vi "Get DTCs From CD and Display.vi"(6 "DTCs":refnum<vi>, 7 "To Top (T)":bool=TRUE, 8 "error in (no error)":errorcluster, 9 "Addresses":refnum<vi>, 10 "Lookup Table In":variant, 11 "connection info":T3) -> (0 "error out":errorcluster, 2 "Lookup Table Out":variant, 3 "connection info":T3, 4 "Error Array":T1[](array[typedef]))   [LabVIEW 2015, in "J1939 Addon Shared.lvlib"]
uses:
  J1939 Addon Shared.lvlib
  <vilib>/NI/STM/TCP/TCP Connection Info.ctl
  <vilib>/NI/STM/SubVIs/MetaDataElement.ctl
  Types/Error Cluster.ctl
  Types/Error Types.ctl
  <vilib>/Utility/miscctls.llb/LVRowAndColumnUnsignedTypeDef.ctl
  <vilib>/NI/STM/NI STM.lvlib
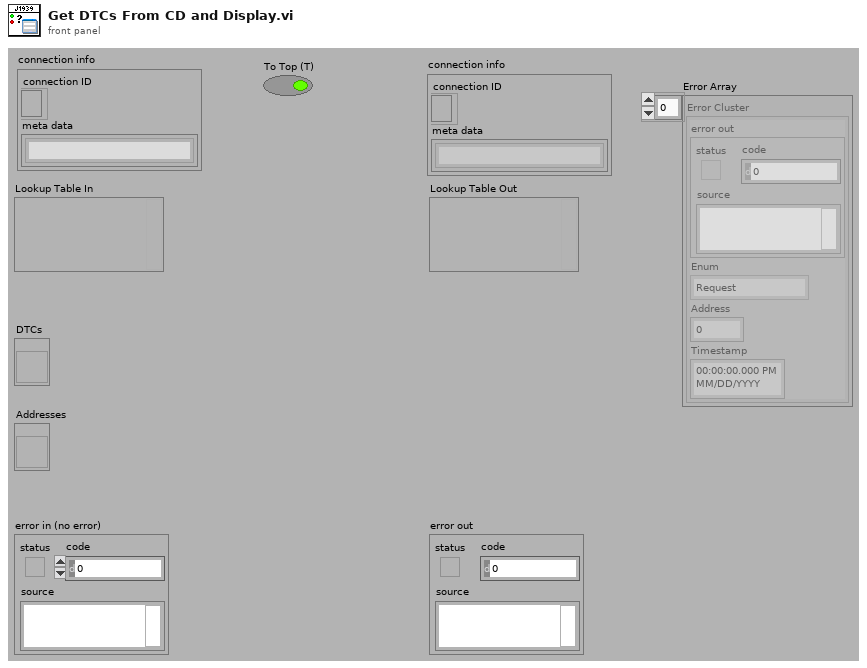
[diagram p1: front panel]
types:
  T1 = typedef "J1939 Addon Shared.lvlib/Error Cluster.ctl" = cluster{"error out":errorcluster, "Enum":T2, "Address":u8, "Timestamp":timestamp}
  T2 = typedef "J1939 Addon Shared.lvlib/Error Types.ctl" = enum16{"Request", "RAW Generation", "Clear Active DTCs", "Clear Previous DTCs", "Addresses", "TLAs", "Get Active DTCs", "Get Previous DTCs"}
  T3 = typedef "NI STM.lvlib/TCP Connection Info.ctl" = cluster{"connection ID":refnum<k5>, "meta data":T4[]}
  T4 = typedef "NI STM.lvlib/MetaDataElement.ctl" = string
  T5 = typedef "J1939 Addon Shared.lvlib/Address Parse Tree Cluster.ctl" = cluster{"Parent Selection":string, "Address Selection":string, "CMD Selection":string}
  T6 = typedef "J1939 Addon Shared.lvlib/Convert DTCs Cluster.ctl" = cluster{"Lamps":cluster{"Protect Lamp":u8, "Amber Warning":u8, "Red Stop":u8, "Malfunction Indicator":u8}, "DTCs":cluster{"SPN":u32, "FMI":u8, "Occurrance":u8}[], "Active?":bool, "Address":u8, "timestamp":timestamp}
  T7 = typedef "LVRowAndColumnUnsignedTypeDef.ctl" = cluster{"Row":u32, "Column":u32}
  T8 = cluster{"Protect Lamp":u8, "Amber Warning":u8, "Red Stop":u8, "Malfunction Indicator":u8}
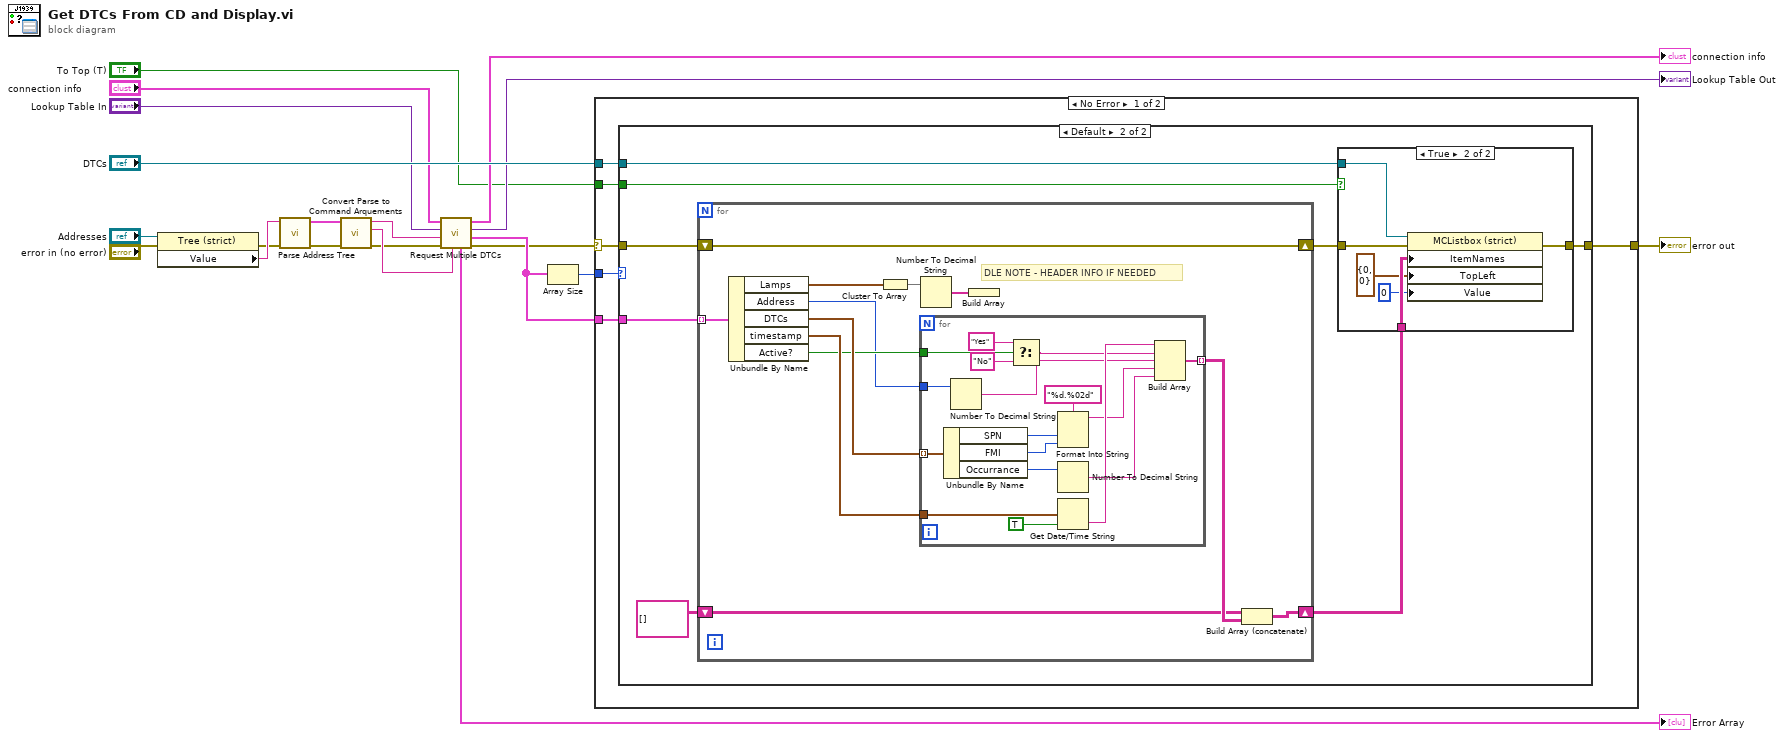
[diagram p0: block diagram]
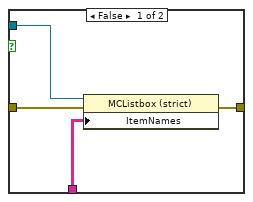
[diagram p3: hidden frame]
diagram:
  n1 = property on="Property Node" class="Tree (strict)"(reference="Addresses", error in="error in (no error)") -> (error out=w14:errorcluster, "Value"=w15:string)  [unwired: 1 out]
  n2 = call "Parse Address Tree.vi"("error in"=w14, "Address Selection"=w15) -> ("error out"=w5:errorcluster, "Address Parsed Tree"=w16:T5)  [unwired: 8 in]
  n3 = call "Convert Parse to Command Arquements.vi"("error in (no error)"=w5, "Address Parsed Tree"=w16) -> ("error out"=w4:errorcluster, "Type"=w10:string, "Address"=w9:string)  [unwired: 7 in]
  n4 = call "Request Multiple DTCs.vi"("Command"=w10, "error in"=w4, "Address"=w9, "Lookup Table"="Lookup Table In", "connection info"="connection info") -> ("error out"=w2:errorcluster, "Responses"=w7:T6[], "Lookup Table Out"=→"Lookup Table Out":variant, "connection info"=→"connection info":T3, "Error Array"=→"Error Array":T1[])  [unwired: 2 in]
  n5 = Array Size(array=w7) -> (size(s)=w8:i32)
  n6 = case shown="No Error" w2 {
    selector: w2 -> [w23 w75]
    tunnel: "DTCs" -> [w26 _]
    tunnel: [w25 w75] -> w17
    tunnel: w8 -> [w24 _]
    tunnel: w7 -> [w22 _]
    tunnel: "To Top (T)" -> [w21 _]
    frame No Error {
      n7 = case shown="Default" w24 {
        tunnel: w23 -> [w27 w29]
        tunnel: w26 -> [_ w33]
        tunnel: [w27 w30] -> w25
        tunnel: w22 -> [_ w35]
        tunnel: w21 -> [_ w28]
        frame 0 {
        }
        frame Default {
          n8 = for {
            tunnel: w35 -> [w48] mode=indexing
            shift-right: [w52] -> w31
            shift-left: w29 -> [w52]
            shift-right: [w50] -> w32
            shift-left: string[][] [] -> [w49]
            # "DLE NOTE - HEADER INFO IF NEEDED"
            n9 = Unbundle By Name(w48) -> ("Lamps"=w54:T8, "Address"=w46:u8, "DTCs"=w57:cluster{"SPN":u32, "FMI":u8, "Occurrance":u8}[], "timestamp"=w53:timestamp, "Active?"=w47:bool)
            n10 = Cluster To Array(cluster=w54) -> (array=w55:u8[])
            n11 = for {
              tunnel: w53 -> [w70]
              tunnel: w57 -> [w74] mode=indexing
              tunnel: [w64] -> w51 mode=indexing
              tunnel: w47 -> [w63]
              tunnel: w46 -> [w59]
              n12 = Unbundle By Name(w74) -> ("SPN"=w73:u32, "FMI"=w72:u8, "Occurrance"=w66:u8)
              n13 = Number To Decimal String(number=w59) -> (decimal integer string=w58:string)  [unwired: 1 in]
              n14 = Select(t="Yes" ("format string"), s=w63, f="No" ("format string")) -> (s? t:f=w62:string)
              n15 = Format Into String(format string="%d.%02d", w73, w72) -> (resulting string=w67:string)  [unwired: 2 in, 1 out]
              n16 = Number To Decimal String(number=w66) -> (decimal integer string=w65:string)  [unwired: 1 in]
              n17 = Get Date/Time String(seconds (now)=w70, want seconds? (F)=TRUE) -> (time string=w68:string)  [unwired: 1 in, 1 out]
              n18 = Build Array(w68, w62, w58, w67, w65) -> (w64:string[])
            }
            n19 = Number To Decimal String(number=w55) -> (decimal integer string=w56:string[])  [unwired: 1 in]
            n20 = Build Array(w56) -> ()  [unwired: 1 out]
            n21 = Build Array (concatenate)(w49, w51) -> (w50:string[][])
          }
          n22 = case shown="True" w28 {
            tunnel: w33 -> [w36 w45]
            tunnel: w32 -> [w38 w44]
            tunnel: w31 -> [w37 w43]
            tunnel: [w39 w42] -> w30
            frame False {
              n23 = property on="Property Node" class="MCListbox (strict)"(reference=w36, error in=w37, "ItemNames"=w38) -> (error out=w39:errorcluster)  [unwired: 1 out]
            }
            frame True {
              n24 = property on="Property Node" class="MCListbox (strict)"(reference=w45, error in=w43, "ItemNames"=w44, "TopLeft"=T7 {"Row"=0, "Column"=0} ("Top Left Visible Cell"), "Value"=0) -> (error out=w42:errorcluster)  [unwired: 1 out]
            }
          }
        }
      }
    }
    frame Error {
    }
  }
  "error out" <- w17
